vi "niRFUtil MASMT 1D Cross Correlation (CSG, SGL).vi"(6 "normalization":i32(ring) items=["None", "Unbiased", "Biased"], 8 "error in (no error)":errorcluster, 9 "algorithm":i32(ring)=1 items=["Direct", "Frequency Domain"], 10 "Y":sgl[](array[numeric]), 11 "X":csg[](array[numeric])) -> (0 "error out":errorcluster, 3 "Rxy":csg[](array[numeric]))   [LabVIEW 2015, in "niRFUtil.lvlib"]
doc: "Computes the cross correlation of the input sequences <B>X</B> and <B>Y</B>."
uses:
  niRFUtil.lvlib
  Utilities/niRFMASMT_FFT.dll
panel:
  out "FreqWorkH":csg[](array[numeric])
  out "WorkH":sgl[](array[numeric])
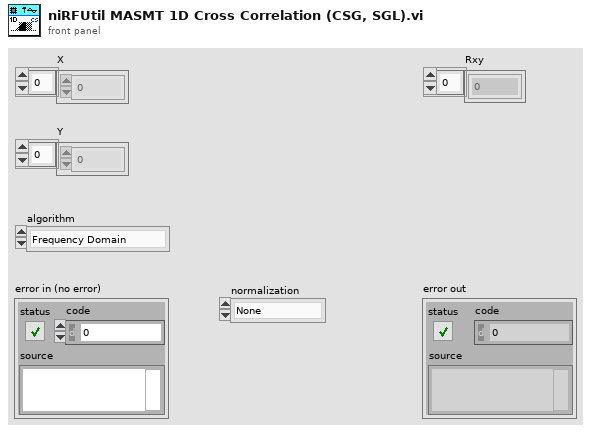
[diagram p1: front panel]
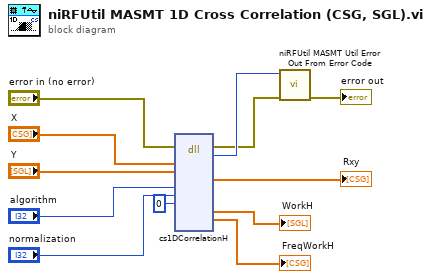
[diagram p0: block diagram]
diagram:
  n1 = dll-call lib="C:/Perforce/semoore-sales/Customers/NATI-3813/Noise Floor/LV Filters/ParallelComplexFilterRFUtil/niRFUtil/MASMT/Utilities/niRFMASMT_FFT.*" fn="cs1DCorrelationH"(error in="error in (no error)", "X"="X", "Y"="Y", "domain"="algorithm", "norm"="normalization", "step"=0) -> (error out=w7:errorcluster, "error"=w9:i32, "Rxy"=→"Rxy":csg[], "txWorkH"=→"WorkH":sgl[], "FreqWorkH"=→"FreqWorkH":csg[])  [unwired: 12 in, 1 out]
  n2 = call "niRFUtil MASMT Util Error Out From Error Code.vi"("error in (no error)"=w7, "error code"=w9) -> ("error out"=→"error out":errorcluster)  [unwired: 9 in]
